vi "Find Instrument Queue.vi"(8 "error in":errorcluster, 10 "Instrument":string, 11 "Launcher in":refnum<class "Launcher.lvclass">) -> (0 "error out":errorcluster, 2 "Queue":refnum<class "Message Enqueuer.lvclass">, 3 "Launcher out":refnum<class "Launcher.lvclass">)   [LabVIEW 2019, in "Launcher.lvlib" / "Launcher.lvclass"]
uses:
  Library/Launcher.lvclass
  builds/Engine/Actor Framework.lvlibp/1abvi3w/vi.lib/ActorFramework/Message Enqueuer/Message Enqueuer.lvclass
  Library/Launcher.lvclass/Launcher.ctl
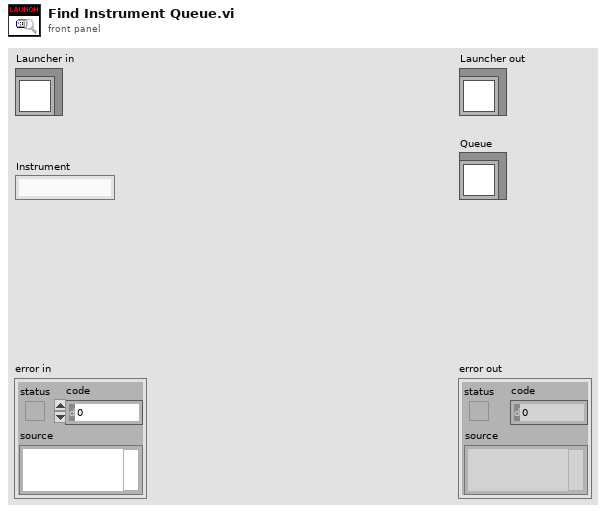
[diagram p1: front panel]
types:
  T1 = cluster{"Identifier":string, "Queue":refnum<class "Message Enqueuer.lvclass">}[]
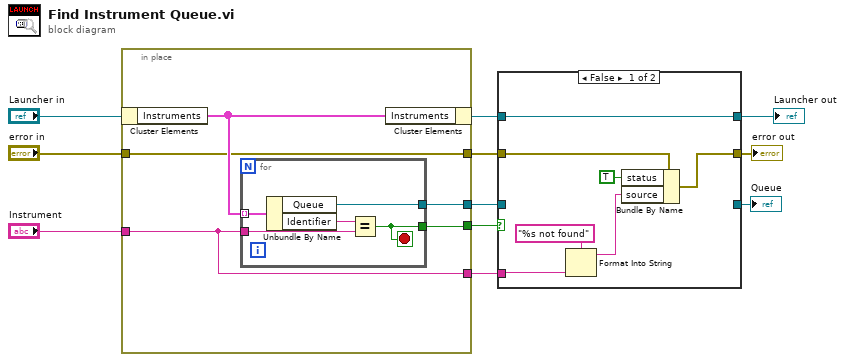
[diagram p0: block diagram]
diagram:
  n1 = in-place {
    in-place-border: "Instrument" -> [w12]
    in-place-border: [w15] -> w8
    in-place-border: [w14] -> w7
    in-place-border: "error in" -> [w13]
    in-place-border: [w13] -> w10
    in-place-border: [w12] -> w11
    n2 = in-place-cluster #1("Launcher in") -> ("Instruments"=w16:T1)
    n3 = for {
      tunnel: w16 -> [w21] mode=indexing
      tunnel: w12 -> [w19]
      tunnel: [w18] -> w15
      tunnel: [w17] -> w14
      stop <- w17 stop-if-true
      n4 = Unbundle By Name(w21) -> ("Queue"=w18:refnum<class "Message Enqueuer.lvclass">, "Identifier"=w20:string)
      n5 = Equal?(x=w20, y=w19) -> (x = y?=w17:bool)
    }
    n6 = in-place-cluster #1("Instruments"=w16) -> (w9:refnum<class "Launcher.lvclass">)
  }
  n7 = case shown="False" w7 {
    tunnel: w8 -> [_ w31]
    tunnel: [_ w31] -> w1
    tunnel: w9 -> [w28 w30]
    tunnel: [w28 w30] -> w5
    tunnel: w10 -> [w27 w29]
    tunnel: [w26 w29] -> w3
    tunnel: w11 -> [w24 _]
    frame False {
      n8 = Format Into String(format string="%s not found", w24) -> (resulting string=w22:string)  [unwired: 2 in, 1 out]
      n9 = Bundle By Name(cluster=w27, "status"=TRUE, "source"=w22) -> (w26:errorcluster)
    }
    frame True {
    }
  }
  "error out" <- w3
  "Launcher out" <- w5
  "Queue" <- w1
